vi "Load Subclasses From Relative Paths File.vi"(8 "error in":errorcluster, 9 "Reference Class Path":path, 10 "Class Relative Paths Path":path, 11 "Caller Enqueuer":refnum<class "Message Enqueuer.lvclass">) -> (0 "error out":errorcluster, 1 "Class Array":refnum<class>[](array[class]), 2 "Class Names":string[](array[string]), 3 "Classes Map":T1)   [LabVIEW 2023, in "Class Loader.lvlib" / "Class Loader.lvclass"]
uses:
  Class Loader.lvclass
  <vilib>/ActorFramework/Message Enqueuer/Message Enqueuer.lvclass
  Class Loader Interfaces/Class Loader Interfaces Messages/Class Loading Progress Msg/Class Loading Progress Msg.lvclass/Class Loading Progress Msg.ctl
  <vilib>/ActorFramework/Message Enqueuer/Message Enqueuer.lvclass/Message Enqueuer.ctl
  <vilib>/ActorFramework/Message Enqueuer/Enqueue.vi
  Class Loader Interfaces/Class Loader Interfaces Messages/Class Loading Progress Msg/Class Loading Progress Msg.lvclass
  C:/Program Files/National Instruments/LabVIEW 2023/vi.lib/ActorFramework/Message/Message.lvclass
  <resource>/AFDebug/Generate Trace for Message.vi
  <vilib>/ActorFramework/Message Priority Queue/Priority Enqueue.vi
  Class Loader.lvclass/Class Loader.ctl
  Class Details.ctl
  ced2505d-d48f-485f-802f-01d2a2dbf5ba.vi
  Classes Map.ctl
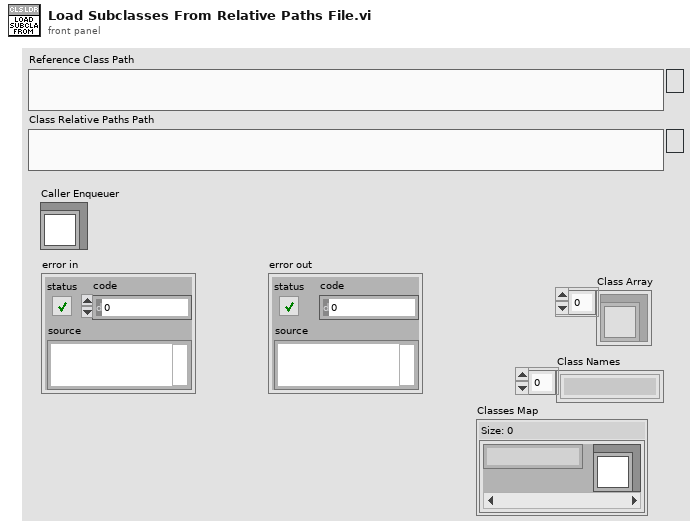
[diagram p1: front panel]
types:
  T1 = typedef "Class Loader.lvlib/Class Loader.lvclass/Classes Map.ctl" = map{string, refnum<class>}
  T2 = enum16{"open", "replace", "create", "open or create", "replace or create", "replace or create with confirmation"}
  T3 = typedef "Class Loader.lvlib/Class Loader.lvclass/Class Details.ctl" = cluster{"Class Name":string, "Class":refnum<class>}
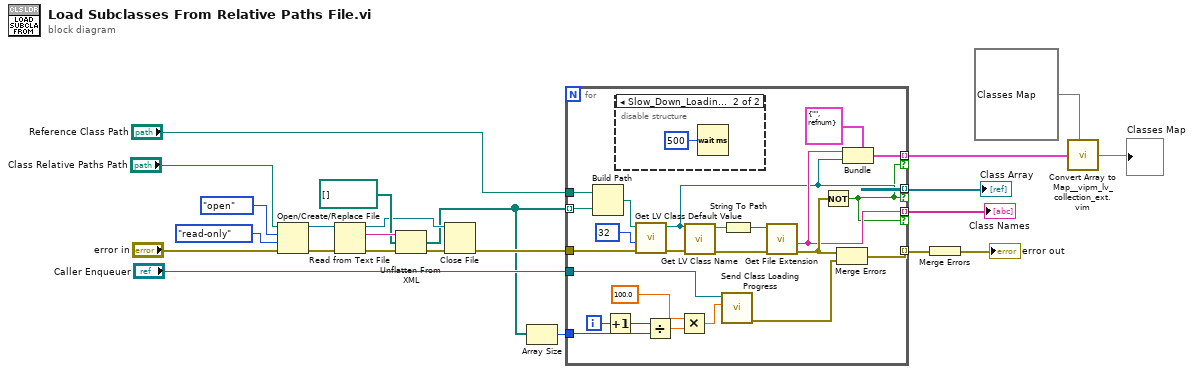
[diagram p0: block diagram]
diagram:
  n1 = Open/Create/Replace File(file path (use dialog)="Class Relative Paths Path", error in="error in", operation (0:open)=T2."open", access (0:read/write)=enum16{"read/write", "read-only", "write-only"}."read-only") -> (refnum out=w19:refnum<file>, error out=w20:errorcluster)  [unwired: 2 in, 1 out]
  n2 = Read from Text File(file (use dialog)=w19, error in=w20) -> (refnum out=w14:refnum<file>, text=w18:string, error out=w16:errorcluster)  [unwired: 2 in, 1 out]
  n3 = Unflatten From XML(xml string=w18, type=path[] [], error in (no error)=w16) -> (value=w5:path[], error out=w15:errorcluster)
  n4 = Close File(refnum=w14, error in=w15) -> (error out=w11:errorcluster)  [unwired: 1 out]
  n5 = Array Size(array=w5) -> (size(s)=w4:i32)
  n6 = for {
    tunnel: w5 -> [w46] mode=indexing
    tunnel: [w35] -> w13 mode=indexing if=w33
    tunnel: "Reference Class Path" -> [w47]
    tunnel: w11 -> [w43]
    tunnel: [w25] -> w10 mode=indexing
    tunnel: [w36] -> w8 mode=indexing if=w33
    tunnel: [w34] -> w2 mode=indexing if=w33
    tunnel: "Caller Enqueuer" -> [w26]
    tunnel: w4 -> [w30]
    i -> [w32]
    n7 = Build Path(base path=w47, name or relative path=w46) -> (appended path=w44:path)
    n8 = Increment(x=w32) -> (x+1=w31:i32)
    n9 = disable-structure shown="Slow_Down_Loading==True" {
      frame condition #0 {
      }
      frame condition #1 (active) {
        n10 = Wait (ms)(milliseconds to wait=u32 500) -> ()  [unwired: 1 out]
      }
    }
    n11 = call <vilib>:"Get LV Class Default Value.vi"("error in (no error)"=w43, "options"=u32 32, "class path"=w44) -> ("error out"=w39:errorcluster, "object"=w35:refnum<class>)  [unwired: 7 in]
    n12 = Divide(x=w31, y=w30) -> (x/y=w29:dbl)
    n13 = Multiply(x=100.0, y=w29) -> (x*y=w27:dbl)
    n14 = call <vilib>:"Get LV Class Name.vi"("error in (no error)"=w39, "object"=w35) -> ("error out"=w42:errorcluster, "class name"=w40:string)  [unwired: 8 in]
    n15 = call "Send Class Loading Progress.vi"("Progress (%)"=w27, "Message Enqueuer"=w26) -> ("error out"=w24:errorcluster)  [unwired: 8 in, 1 out]
    n16 = String To Path(string=w40) -> (path=w41:path)
    n17 = call <vilib>:"Get File Extension.vi"("error in (no error)"=w42, "file"=w41) -> ("error out"=w38:errorcluster, "filename without extension"=w36:string)  [unwired: 5 in, 3 out]
    n18 = Not(x=w38) -> (.not. x?=w33:bool)
    n19 = Merge Errors(w38, w24) -> (w25:errorcluster)
    n20 = Bundle(cluster=T3 {"Class Name"="", "Class"=refnum} ("Class Details"), "Class Name"=w36, "Class"=w35) -> (w34:T3)
  }
  "Class Array" <- w13
  "Class Names" <- w8
  n21 = Merge Errors(w10) -> (→"error out":errorcluster)
  n22 = call "Convert Array to Map__vipm_lv_collection_ext.vim"("map type (optional)"=T1 {} ("Classes Map"), "array"=w2) -> ("map"=→"Classes Map":T1)  [unwired: 5 in]
